vi "Convert 2D Array to Dictionary.vi"(0 "CSV Data":string[][](array[string]), 11 "Error in":errorcluster caption="Error in (no error)") -> (4 "Dictionary out":refnum<class "Dictionary.lvclass">, 8 "Headers":string[](array[string]), 15 "Error out":errorcluster)   [LabVIEW 2018]
doc: "Convert 2D array to Dictionary\n\nKåre Juul Kirkegaard\nGPower\n7/4 2019"
uses:
  <vilib>/GPower/Dictionary/Library/Dictionary Class/Dictionary.lvclass
  758e3b9e-21e9-431f-9e65-975b05c0325a.vi
  <vilib>/GPower/Dictionary/Library/Dictionary Class/Set/Set Or Append Value.vi
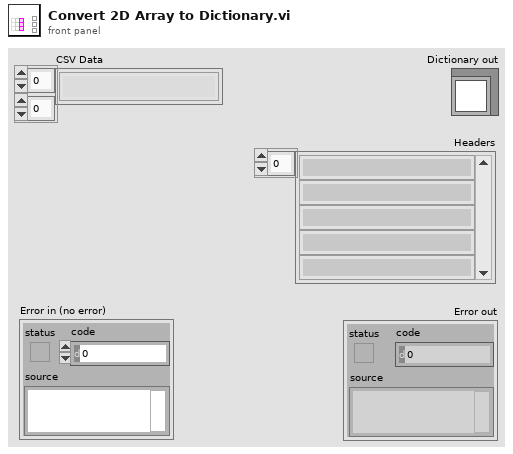
[diagram p1: front panel]
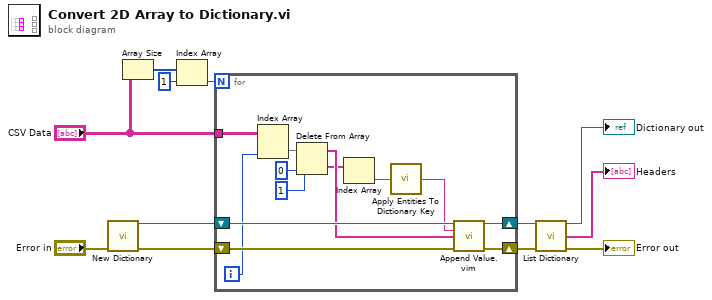
[diagram p0: block diagram]
diagram:
  n1 = call <vilib>:"New Dictionary.vi"("Error in"="Error in") -> ("New Dictionary"=w10:refnum<class "Dictionary.lvclass">, "Error out"=w12:errorcluster)  [unwired: 13 in]
  n2 = Array Size(array="CSV Data") -> (size(s)=w9:i32[])
  n3 = Index Array(array=w9, index=1) -> (element=w7:i32)
  n4 = for {
    N: w7 -> [_]
    tunnel: "CSV Data" -> [w17]
    shift-right: [w19] -> w4
    shift-left: w12 -> [w25]
    shift-right: [w18] -> w6
    shift-left: w10 -> [w24]
    i -> [w15]
    n5 = Index Array(array=w17, index (col)=w15) -> (element=w16:string[])  [unwired: 1 in]
    n6 = Delete From Array(array=w16, length=1, index=0) -> (deleted portion=w20:string[], array with subset deleted=w21:string[])
    n7 = Index Array(array=w20) -> (element=w14:string)  [unwired: 1 in]
    n8 = call <vilib>:"Apply Entities To Dictionary Key.vi"("Clear Dictionary Key"=w14) -> ("Encoded Dictionary Key"=w13:string)
    n9 = call "Append Value.vim"("Dictionary in"=w24, "Requested Key Path"=w13, "Value"=w21, "Error in"=w25) -> ("Dictionary out"=w18:refnum<class "Dictionary.lvclass">, "Error out"=w19:errorcluster)  [unwired: 9 in, 1 out]
  }
  n10 = call <vilib>:"List Dictionary.vi"("Dictionary in"=w6, "Error in"=w4) -> ("Dictionary out"=→"Dictionary out":refnum<class "Dictionary.lvclass">, "Keys"=→"Headers":string[], "Error out"=→"Error out":errorcluster)  [unwired: 11 in]
